vi "UserMarkBadResultsZ.vi"(5 "Log file":path=path "nologfile", 6 "ID summary":T1(array[cluster]), 7 "Database":T2={"DB name"="zaop", "UID"="jdennis", "password"=""}) -> (0 "error out":errorcluster)   [LabVIEW 2016]
doc: "This program displays measurement results when the end of a list of measurements is reached. The user can modify \"data usable\", and after \"Continue\" is clicked, the changes are made in the databas. The display shows measurement setting and result IDs (measSetId and measResId), errors or warnings found, and the current status of the \"data usable\" field."
uses:
  type def/Database.ctl
panel:
  in  "Continue":bool
  out "bad resId":cluster{"measResId":i32, "status":bool}[](array[cluster]) caption="measResId"
  in  "Mark data":T3(array[cluster])
  in  "error in (no error)":errorcluster
  # "Any results which had errors or warnings are listed below. Check the summary at right, and select yes or no under \"Data usable?\" Then press Continue"
  # "Program constants"
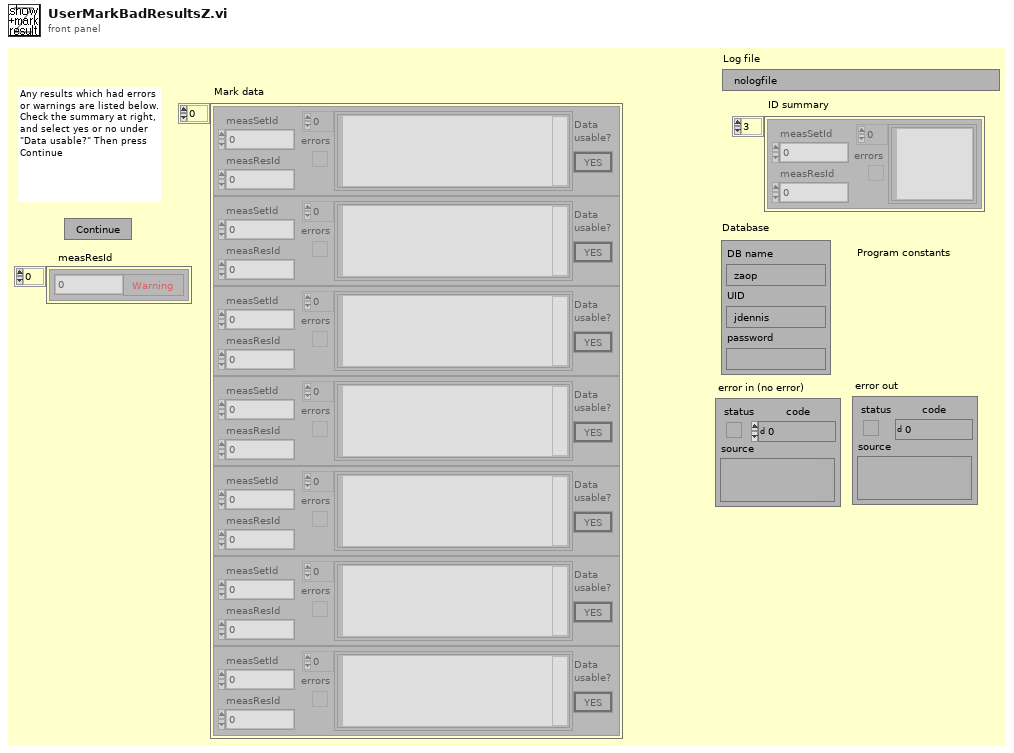
[diagram p1: front panel]
types:
  T1 = cluster{"measSetId":i32, "measResId":i32, "errors":string[], "status":bool}[]
  T2 = typedef "Database.ctl" = cluster{"DB name":string, "UID":string, "password":string}
  T3 = cluster{"measSetId":i32, "measResId":i32, "errors":string[], "status":bool, "Data\nusable?":bool}[]
  T4 = cluster{"measSetId":i32, "measResId":i32, "errors":string[], "status":bool, "Data\nusable?":bool}
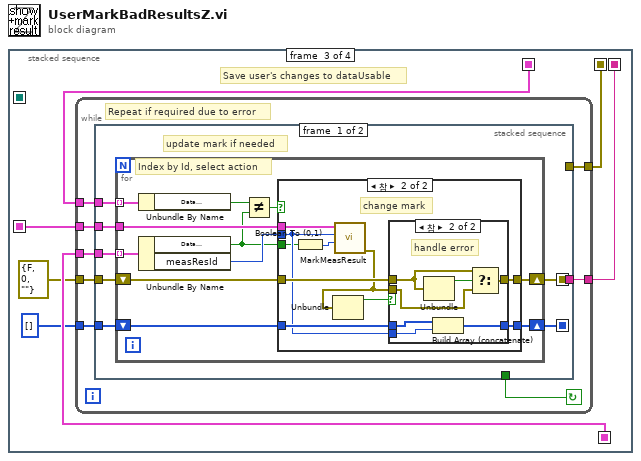
[diagram p0: block diagram]
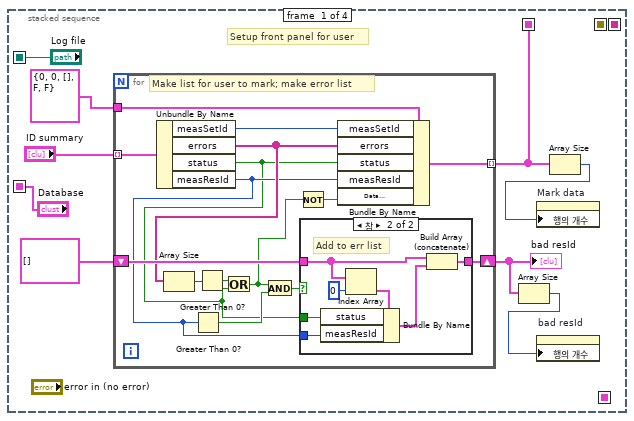
[diagram p2: hidden frame]
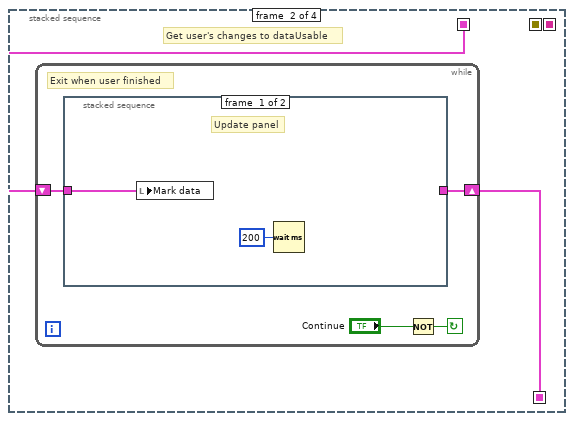
[diagram p4: hidden frame]
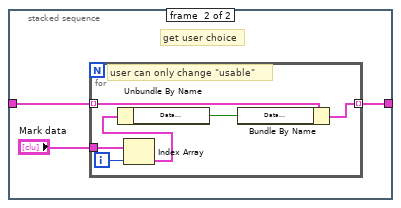
[diagram p5: hidden frame]
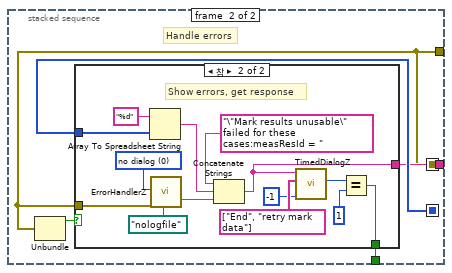
[diagram p8: hidden frame]
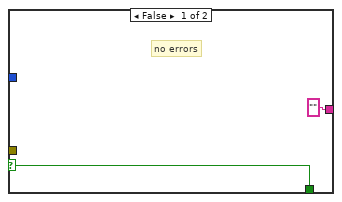
[diagram p9: hidden frame]
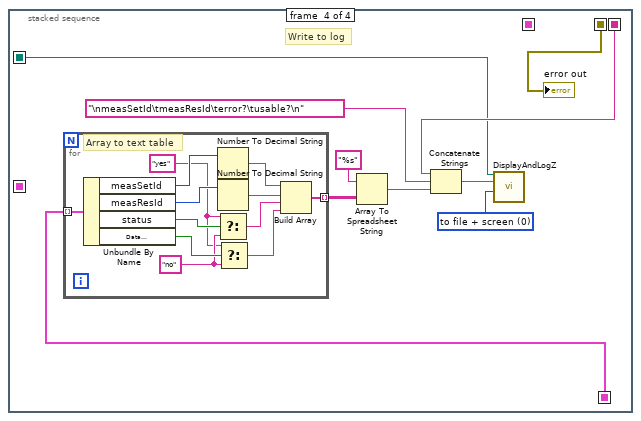
[diagram p10: hidden frame]
diagram:
  n1 = stacked-sequence {
    seq-local: [_ w34 _ _] -> [_ _ w56 w133]
    seq-local: ["Database" _ _ _] -> [_ _ w55 _]
    seq-local: [w3 _ _ _] -> [_ w33 w50 _]
    seq-local: [_ _ w52 _] -> [_ _ _ w134]
    seq-local: ["Log file" _ _ _] -> [_ _ _ w126]
    seq-local: [_ _ w51 _] -> [_ _ _ w125]
    frame #0 {
      # "Setup front panel for user"
      n2 = for {
        tunnel: "ID summary" -> [w24] mode=indexing
        shift-right: [w20] -> w5
        shift-left: cluster{"measResId":i32, "status":bool}[] [] ("bad resId") -> [w19]
        tunnel: T4 {"measSetId"=0, "measResId"=0, "errors"=[], "status"=FALSE, "Data\nusable?"=FALSE} ("Cluster") -> [w17]
        tunnel: [w12] -> w3 mode=indexing
        # "Make list for user to mark; make error list"
        n3 = Unbundle By Name(w24) -> ("measSetId"=w16:i32, "errors"=w15:string[], "status"=w11:bool, "measResId"=w14:i32)
        n4 = Array Size(array=w15) -> (size(s)=w22:i32)
        n5 = Greater Than 0?(x=w14) -> (x > 0?=w23:bool)
        n6 = Greater Than 0?(x=w22) -> (x > 0?=w21:bool)
        n7 = Or(x=w21, y=w11) -> (x .or. y?=w10:bool)
        n8 = And(x=w10, y=w23) -> (x .and. y?=w18:bool)
        n9 = Not(x=w10) -> (.not. x?=w13:bool)
        n10 = case shown="참" w18 {
          tunnel: [w25 w32] -> w20
          tunnel: w19 -> [w25 w27]
          tunnel: w11 -> [_ w31]
          tunnel: w14 -> [_ w30]
          frame False {
            # "no error"
          }
          frame True {
            # "Add to err list"
            n11 = Index Array(array=w27, index=0 ("Index")) -> (element=w26:cluster{"measResId":i32, "status":bool})
            n12 = Bundle By Name(cluster=w26, "status"=w31, "measResId"=w30) -> (w29:cluster{"measResId":i32, "status":bool})
            n13 = Build Array (concatenate)(w27, w29) -> (w32:cluster{"measResId":i32, "status":bool}[])
          }
        }
        n14 = Bundle By Name(cluster=w17, "measSetId"=w16, "errors"=w15, "status"=w11, "measResId"=w14, "Data\nusable?"=w13) -> (w12:T4)
      }
      "bad resId" <- w5
      n15 = Array Size(array=w5) -> (size(s)=w4:i32)
      n16 = property on="bad resId" class="Arr (엄격한)"("행의 개수"=w4) -> ()  [unwired: 2 in, 2 out]
      n17 = Array Size(array=w3) -> (size(s)=w2:i32)
      n18 = property on="Mark data" class="Arr (엄격한)"("행의 개수"=w2) -> ()  [unwired: 2 in, 2 out]
    }
    frame #1 {
      # "Get user's changes to dataUsable"
      n19 = while {
        shift-left: w33 -> [w36]
        shift-right: [w35] -> w34
        stop <- w38 continue-if-true
        # "Exit when user finished"
        n20 = stacked-sequence {
          tunnel: w36 -> [w39 w43]
          tunnel: [_ w42] -> w35
          frame #0 {
            # "Update panel"
            n21 = local write "Mark data"(w39) -> ()
            n22 = Wait (ms)(milliseconds to wait=u32 200) -> ()  [unwired: 1 out]
          }
          frame #1 {
            # "get user choice"
            n23 = for {
              tunnel: "Mark data" -> [w45]
              tunnel: w43 -> [w49] mode=indexing
              tunnel: [w48] -> w42 mode=indexing
              i -> [w46]
              # "user can only change \"usable\""
              n24 = Index Array(array=w45, index=w46) -> (element=w44:T4)
              n25 = Unbundle By Name(w44) -> ("Data\nusable?"=w47:bool)
              n26 = Bundle By Name(cluster=w49, "Data\nusable?"=w47) -> (w48:T4)
            }
          }
        }
        n27 = Not(x="Continue") -> (.not. x?=w38:bool)
      }
    }
    frame #2 {
      # "Save user's changes to dataUsable"
      n28 = while {
        tunnel: w50 -> [w57]
        tunnel: [w58] -> w51
        tunnel: [w59] -> w52
        tunnel: errorcluster {"status"=FALSE, "code"=0, "source"=""} ("error in (no error)") -> [w61]
        tunnel: i32[] [] ("Array Constant") -> [w62]
        tunnel: w55 -> [w63]
        tunnel: w56 -> [w64]
        stop <- w60 continue-if-true
        # "Repeat if required due to error"
        n29 = stacked-sequence {
          seq-local: [w66 _] -> [_ w104]
          seq-local: [w67 _] -> [_ w107]
          tunnel: w64 -> [w71 _]
          tunnel: w63 -> [w70 _]
          tunnel: w62 -> [w69 _]
          tunnel: w61 -> [w68 _]
          tunnel: [_ w106] -> w60
          tunnel: [_ w105] -> w59
          tunnel: [_ w104] -> w58
          tunnel: w57 -> [w65 _]
          frame #0 {
            # "update mark if needed"
            n30 = for {
              tunnel: w71 -> [w81] mode=indexing
              tunnel: w70 -> [w82]
              shift-right: [w79] -> w66
              shift-left: w68 -> [w78]
              shift-right: [w77] -> w67
              shift-left: w69 -> [w76]
              tunnel: w65 -> [w75] mode=indexing
              # "Index by Id, select action"
              n31 = Unbundle By Name(w75) -> ("Data\nusable?"=w74:bool)
              n32 = Unbundle By Name(w81) -> ("Data\nusable?"=w72:bool, "measResId"=w80:i32)
              n33 = Not Equal?(x=w74, y=w72) -> (x != y?=w73:bool)
              n34 = case shown="참" w73 {
                tunnel: w82 -> [_ w94]
                tunnel: w80 -> [_ w88]
                tunnel: [w84 w92] -> w79
                tunnel: w78 -> [w84 w91]
                tunnel: [w83 w90] -> w77
                tunnel: w76 -> [w83 w89]
                tunnel: w72 -> [_ w86]
                frame False {
                  # "no change to mark"
                }
                frame True {
                  # "change mark"
                  n35 = Boolean To (0,1)(Boolean=w86) -> (0, 1=w85:i16)
                  n36 = call "MarkMeasResult.vi"("Data useful?"=w85, "measResId"=w88, "Database"=w94) -> ("error out"=w87:errorcluster)  [unwired: 4 in]
                  n37 = Unbundle(w87) -> ("status"=w93:bool)  [unwired: 2 out]
                  n38 = case shown="참" w93 {
                    tunnel: [w96 w100] -> w92
                    tunnel: w91 -> [w96 w102]
                    tunnel: w87 -> [_ w101]
                    tunnel: [w95 w97] -> w90
                    tunnel: w89 -> [w95 w99]
                    tunnel: w88 -> [_ w98]
                    frame False {
                      # "no error"
                    }
                    frame True {
                      # "handle error"
                      n39 = Unbundle(w102) -> ("status"=w103:bool)  [unwired: 2 out]
                      n40 = Build Array (concatenate)(w99, w98) -> (w97:i32[])
                      n41 = Select(t=w102, s=w103, f=w101) -> (s? t:f=w100:errorcluster)
                    }
                  }
                }
              }
            }
          }
          frame #1 {
            # "Handle errors"
            n42 = Unbundle(w104) -> ("status"=w108:bool)  [unwired: 2 out]
            n43 = case shown="참" w108 {
              selector: w108 -> [w110 _]
              tunnel: w104 -> [_ w124]
              tunnel: w107 -> [_ w121]
              tunnel: [w110 w112] -> w106
              tunnel: ["" w111] -> w105
              frame False {
                # "no errors"
              }
              frame True {
                w122 = u16 0 items=["no dialog", "timed OK message", "timed options message"] ("type of dialog (timed opt:2)")
                # "Show errors, get response"
                n44 = Array To Spreadsheet String(array=w121, 3:"%d" ("format string")) -> (spreadsheet string=w118:string)  [unwired: 1 in]
                n45 = call "ErrorHandlerZ.vi"("type of dialog (timed opt:2)"=w122, "error in (no error)"=w124, "Log file"=path "nologfile") -> ("message"=w117:string)  [unwired: 11 in, 5 out]
                n46 = Concatenate Strings("\"Mark results unusable\" failed for these cases:measResId = ", w118, w117) -> (w111:string)
                n47 = call "TimedDialogZ.vi"("dialog sec (60)"=-1, "option list"=string[] ["End", "retry mark data"], "Dialog text"=w111) -> ("selection (timeout -1)"=w113:i32)  [unwired: 6 in]
                n48 = Equal?(x=w113, y=i8 1) -> (x = y?=w112:bool)
              }
            }
          }
        }
      }
    }
    frame #3 {
      w127 = u16 0 items=["to file + screen", "to file", "to screen", "clear screen"] ("action")
      # "Write to log"
      n49 = for {
        tunnel: w133 -> [w146] mode=indexing
        tunnel: [w135] -> w132 mode=indexing
        w141 = "no"
        w140 = "yes"
        # "Array to text table"
        n50 = Unbundle By Name(w146) -> ("measSetId"=w145:i32, "measResId"=w144:i32, "status"=w143:bool, "Data\nusable?"=w142:bool)
        n51 = Number To Decimal String(number=w145) -> (decimal integer string=w139:string)  [unwired: 1 in]
        n52 = Number To Decimal String(number=w144) -> (decimal integer string=w138:string)  [unwired: 1 in]
        n53 = Select(t=w140, s=w143, f=w141) -> (s? t:f=w137:string)
        n54 = Select(t=w140, s=w142, f=w141) -> (s? t:f=w136:string)
        n55 = Build Array(w139, w138, w137, w136) -> (w135:string[])
      }
      n56 = Array To Spreadsheet String(array=w132, 3:"%s" ("format string")) -> (spreadsheet string=w130:string)  [unwired: 1 in]
      n57 = Concatenate Strings(w134, "\nmeasSetId\tmeasResId\terror?\tusable?\n", w130) -> (w128:string)
      n58 = call "DisplayAndLogZ.vi"("Log file"=w126, "message"=w128, "action (0: log+display)"=w127) -> ()  [unwired: 5 in, 1 out]
      "error out" <- w125
    }
  }
